vi "procedura configura potenza BANCO 2.vi"(9 "All Data":T3 {"MISURE ALL"."Cluster READ NI"."AI (4-20mA)"."AI 15" format="%#_6f"; "MISURE ALL"."Cluster READ NI"."AI (4-20mA)"."AI 14" format="%#_6f"; "MISURE ALL"."Cluster READ NI"."AI (4-20mA)"."AI 13" format="%#_6f"; "MISURE ALL"."Cluster READ NI"."AI (4-20mA)"."AI 11" format="%#_6f"; "MISURE ALL"."Cluster READ NI"."AI (4-20mA)"."AI 10" format="%#_6f"; "MISURE ALL"."Cluster READ NI"."AI (4-20mA)"."AI 9" format="%#_6f"; "MISURE ALL"."Cluster READ NI"."AI (4-20mA)"."AI 4" format="%#_6f"; "MISURE ALL"."Cluster READ NI"."AI (4-20mA)"."AI 12" format="%#_6f"; "MISURE ALL"."Cluster READ NI"."AI (4-20mA)"."AI 0" format="%#_6f"; "MISURE ALL"."Cluster READ NI"."AI (4-20mA)"."AI 1" format="%#_6f"; "MISURE ALL"."Cluster READ NI"."AI (4-20mA)"."AI 2" format="%#_6f"; "MISURE ALL"."Cluster READ NI"."AI (4-20mA)"."AI 3" format="%#_6f"; "MISURE ALL"."Cluster READ NI"."AI (4-20mA)"."AI 5" format="%#_6f"; "MISURE ALL"."Cluster READ NI"."AI (4-20mA)"."AI 6" format="%#_6f"; "MISURE ALL"."Cluster READ NI"."AI (4-20mA)"."AI 7" format="%#_6f"; "MISURE ALL"."Cluster READ NI"."AI (4-20mA)"."AI 8" format="%#_6f"; "MISURE ALL"."Cluster READ NI"."AI (0-10V)"."AI 31" format="%#_6f"; "MISURE ALL"."Cluster READ NI"."AI (0-10V)"."AI 30" format="%#_6f"; "MISURE ALL"."Cluster READ NI"."AI (0-10V)"."AI 29" format="%#_6f"; "MISURE ALL"."Cluster READ NI"."AI (0-10V)"."AI 28" format="%#_6f"; "MISURE ALL"."Cluster READ NI"."AI (0-10V)"."AI 27" format="%#_6f"; "MISURE ALL"."Cluster READ NI"."AI (0-10V)"."AI 26" format="%#_6f"; "MISURE ALL"."Cluster READ NI"."AI (0-10V)"."AI 25" format="%#_6f"; "MISURE ALL"."Cluster READ NI"."AI (0-10V)"."AI 24" format="%#_6f"; "MISURE ALL"."Cluster READ NI"."AI (0-10V)"."AI 23" format="%#_6f"; "MISURE ALL"."Cluster READ NI"."AI (0-10V)"."AI 22" format="%#_6f"; "MISURE ALL"."Cluster READ NI"."AI (0-10V)"."AI 21" format="%#_6f"; "MISURE ALL"."Cluster READ NI"."AI (0-10V)"."AI 20" format="%#_6f"; "MISURE ALL"."Cluster READ NI"."AI (0-10V)"."AI 19" format="%#_6f"; "MISURE ALL"."Cluster READ NI"."AI (0-10V)"."AI 18" format="%#_6f"; "MISURE ALL"."Cluster READ NI"."AI (0-10V)"."AI 17" format="%#_6f"; "MISURE ALL"."Cluster READ NI"."AI (0-10V)"."AI 16" format="%#_6f"; "MISURE ALL"."Cluster READ NI"."AI (0-10V)"."AI 15" format="%#_6f"; "MISURE ALL"."Cluster READ NI"."AI (0-10V)"."AI 14" format="%#_6f"; "MISURE ALL"."Cluster READ NI"."AI (0-10V)"."AI 13" format="%#_6f"; "MISURE ALL"."Cluster READ NI"."AI (0-10V)"."AI 11" format="%#_6f"; "MISURE ALL"."Cluster READ NI"."AI (0-10V)"."AI 10" format="%#_6f"; "MISURE ALL"."Cluster READ NI"."AI (0-10V)"."AI 9" format="%#_6f"; "MISURE ALL"."Cluster READ NI"."AI (0-10V)"."AI 4" format="%#_6f"; "MISURE ALL"."Cluster READ NI"."AI (0-10V)"."AI 12" format="%#_6f"; "MISURE ALL"."Cluster READ NI"."AI (0-10V)"."AI 0" format="%#_6f"; "MISURE ALL"."Cluster READ NI"."AI (0-10V)"."AI 1" format="%#_6f"; "MISURE ALL"."Cluster READ NI"."AI (0-10V)"."AI 2" format="%#_6f"; "MISURE ALL"."Cluster READ NI"."AI (0-10V)"."AI 3" format="%#_6f"; "MISURE ALL"."Cluster READ NI"."AI (0-10V)"."AI 5" format="%#_6f"; "MISURE ALL"."Cluster READ NI"."AI (0-10V)"."AI 6" format="%#_6f"; "MISURE ALL"."Cluster READ NI"."AI (0-10V)"."AI 7" format="%#_6f"; "MISURE ALL"."Cluster READ NI"."AI (0-10V)"."AI 8" format="%#_6f"}, 10 "Impostazioni elettriche in":T2, 11 "Stato":string) -> (0 "This VI":refnum<vi>, 2 "Boolean":bool, 3 "stato":string)   [LabVIEW 2019]
uses:
  TypeDef/Cluster MISURE.ctl
  TypeDef/MISURE NM.ctl
  TypeDef/Cluster misure ALL.ctl
  TypeDef/Cluster NI.ctl
  cDAQ_PLC Folder/controls/StatoAO_cdaq.ctl
  cDAQ_PLC Folder/controls/statoDO_Cdaq.ctl
  TypeDef/MISURE WT.ctl
  TypeDef/ClusterRes.ctl
  TypeDef/INTERFACCIA.ctl
  TypeDef/Lista AO sistema.ctl
  TypeDef/DOinterfaccia.ctl
  cDAQ_PLC Folder/ST1200_LIST_IO/STATO PLC 1.ctl
  cDAQ_PLC Folder/ST1200_LIST_IO/Uscite PLC 1.ctl
  cDAQ_PLC Folder/controls/statoAO_plc_1.ctl
  cDAQ_PLC Folder/ST1200_LIST_IO/StatoDO_PLC_1.ctl
  SINUS PENTA SANTERNO/controls/Parametri inverter letti.ctl
  cDAQ_PLC Folder/ST1200_LIST_IO/STATO PLC 2.ctl
  cDAQ_PLC Folder/ST1200_LIST_IO/Uscite PLC 2.ctl
  cDAQ_PLC Folder/controls/statoAO_plc_2.ctl
  cDAQ_PLC Folder/ST1200_LIST_IO/StatoDO_PLC_2.ctl
  cDAQ_PLC Folder/ST1200_LIST_IO/STATO PLC 3.ctl
  cDAQ_PLC Folder/ST1200_LIST_IO/Uscite PLC 3.ctl
  cDAQ_PLC Folder/controls/statoAO_plc_3.ctl
  cDAQ_PLC Folder/ST1200_LIST_IO/StatoDO_PLC_3.ctl
  DCREG/Parametri DCREG letti.ctl
  TypeDef/Impostazioni elettriche.ctl
  TypeDef/Collegamenti_elettrici.ctl
  cDAQ_PLC Folder/cDAQ/SET ARRAY DO.ctl
  cDAQ_PLC Folder/cDAQ/SET SINGLE DO.ctl
  cDAQ_PLC Folder/cDAQ/DO List.ctl
  Global allarmi procedure.vi
panel:
  out "COLLEGAMENTO":T1
  out "Stato 2":string
  out "String":string
  # "CONFIGURAZIONE BANCO 2  (KEB)"
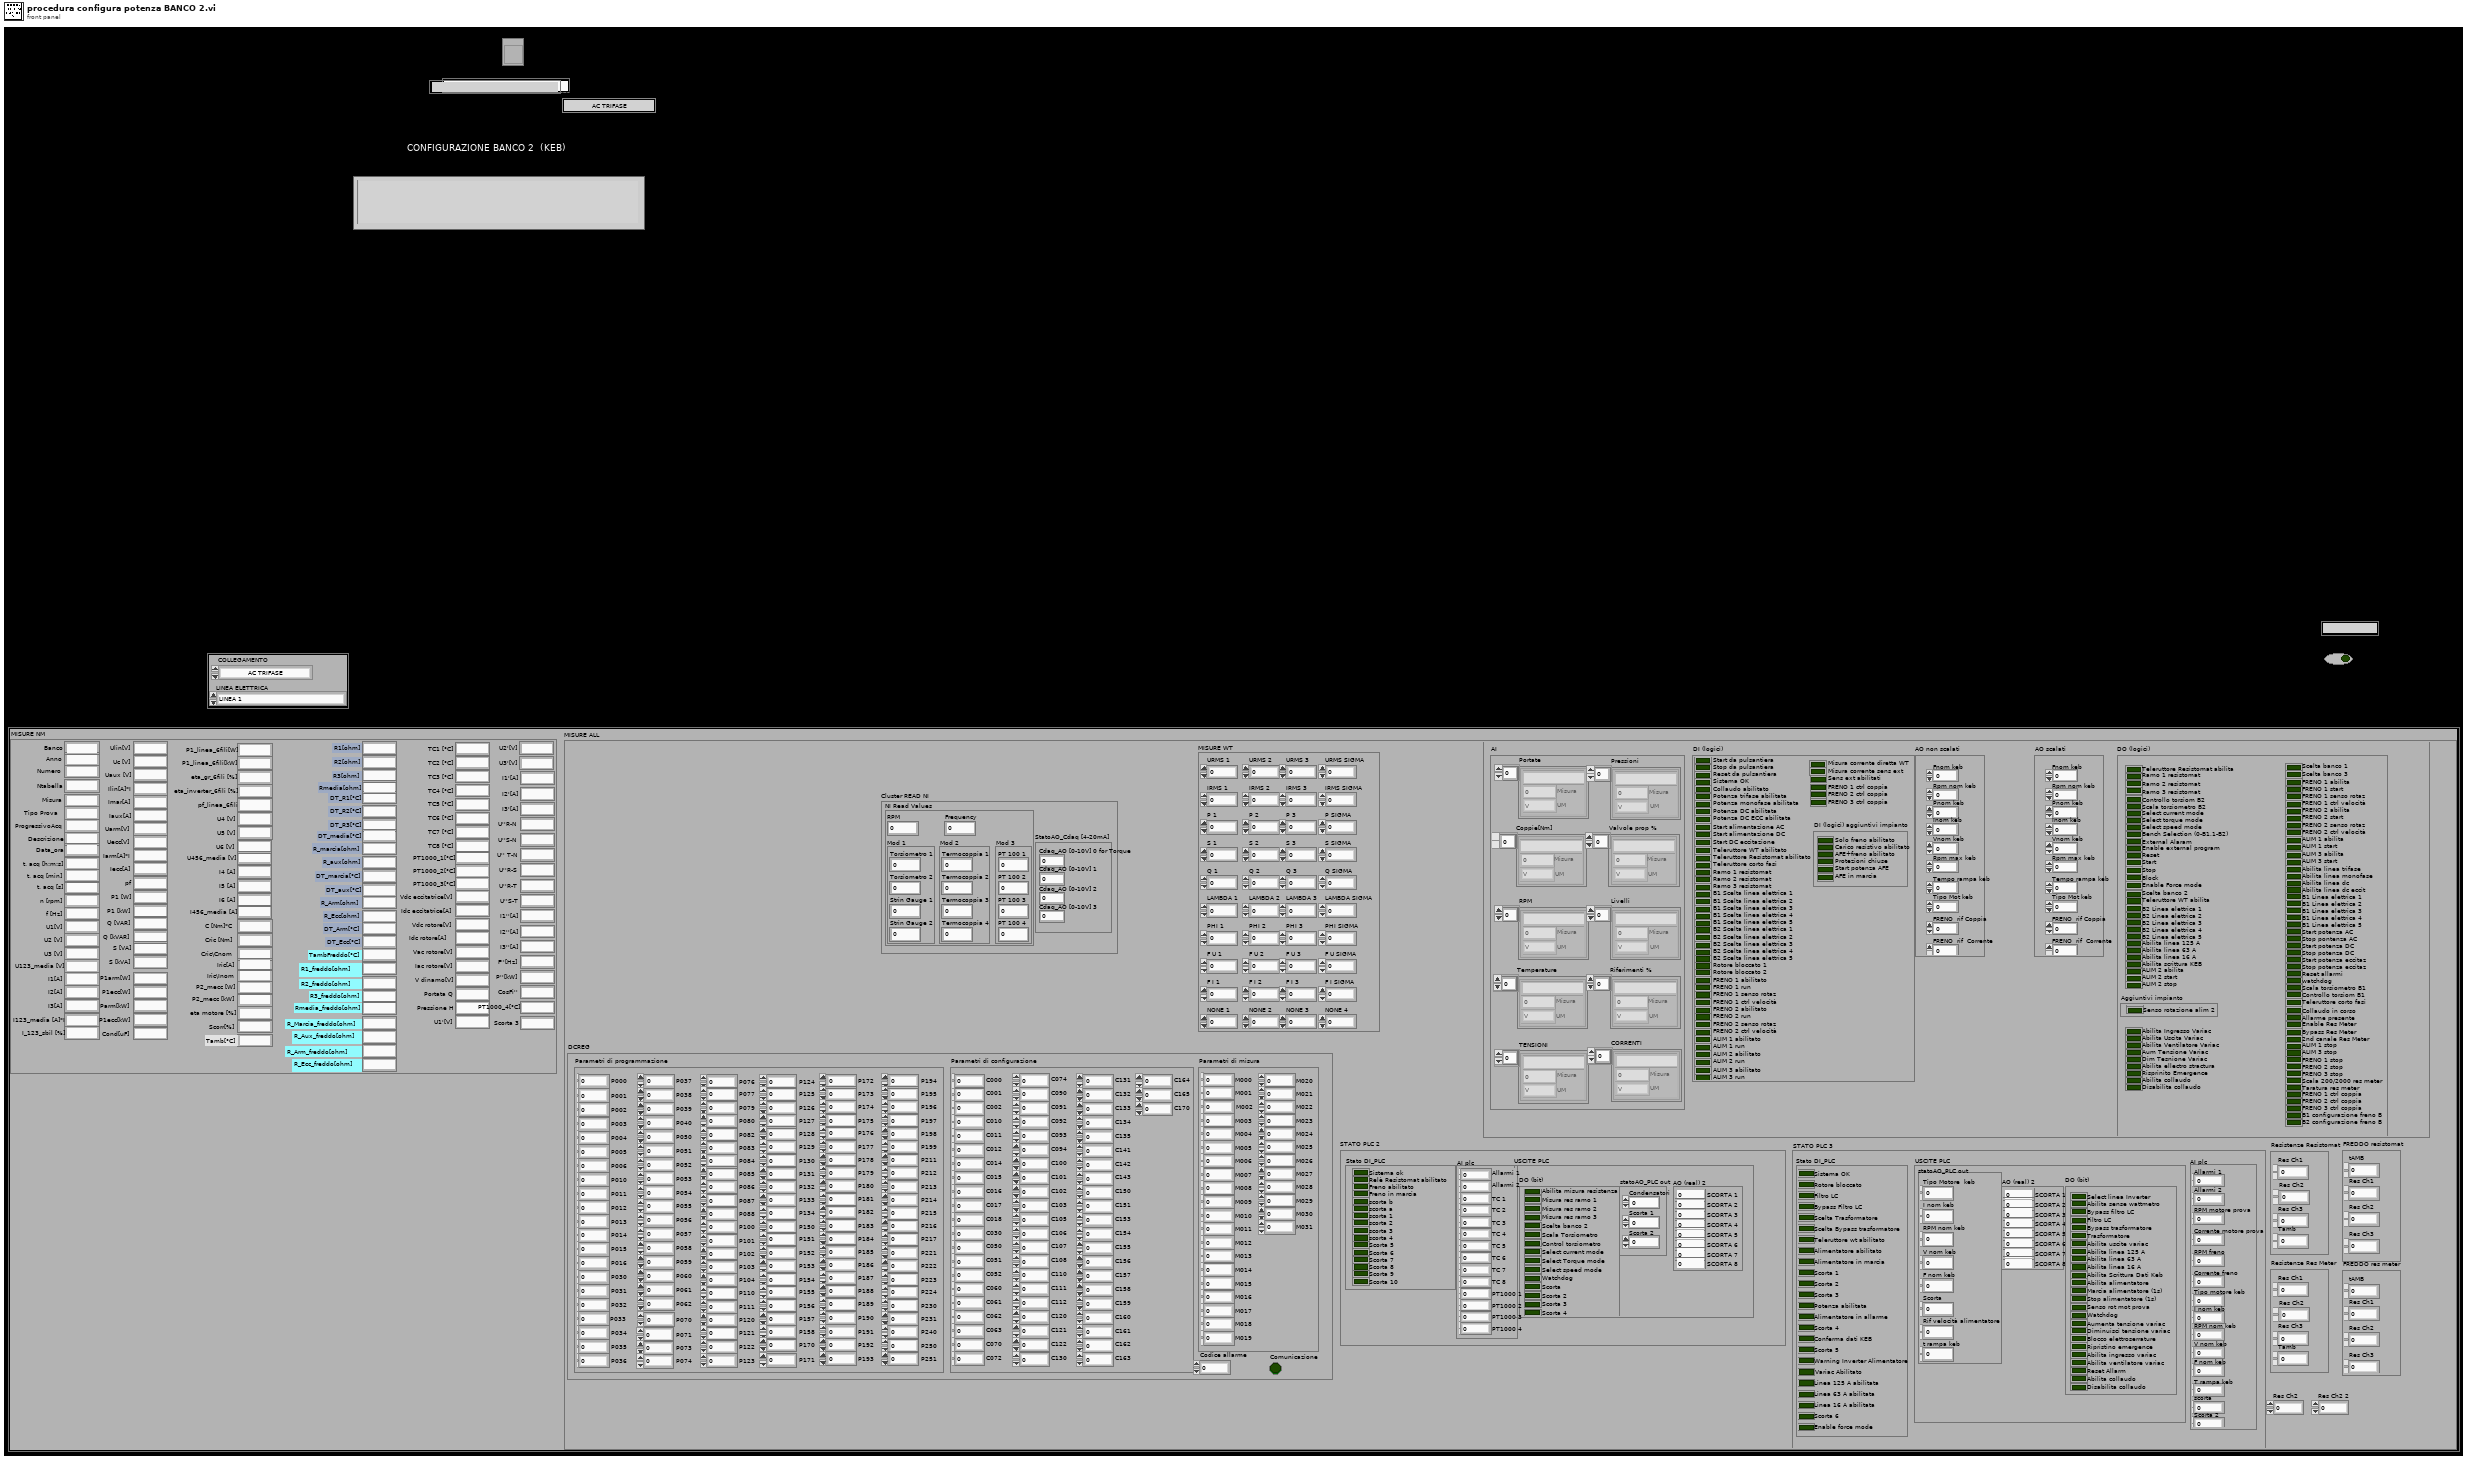
[diagram p1: front panel]
types:
  T1 = typedef "Collegamenti_elettrici.ctl" = enum16{"AC TRIFASE", "AC TRIFASE + FRENO", "AC MONOFASE", "DC CON ECCITAZIONE", "DC CON ECCITAZIONE + FRENO", "DC NO ECCITAZIONE", "DC NO ECCITAZIONE + FRENO", "FRENO TRASC + AFE", "SOLO FRENO", "CARICO RESISTIVO", "GENERICO", "SOLO ACQUISITORE", "SCORTA 4", "SCORTA 5", "SCORTA 6"}
  T2 = typedef "Impostazioni elettriche.ctl" = cluster{"COLLEGAMENTO":T1, "LINEA ELETTRICA":enum16{"LINEA 1", "LINEA 2", "LINEA 3", "LINEA 4", "LINEA 5"}}
  T3 = typedef "Cluster MISURE.ctl" = cluster{"MISURE NM":T4, "MISURE ALL":T5}
  T4 = typedef "MISURE NM.ctl" = cluster{"Banco":string, "Anno":string, "Numero":string, "Ntabella":string, "Misura":string, "Tipo Prova":string, "ProgressivoAcq":string, "Descrizione":string, "Data_ora":string, "t. acq [h:m:s]":string, "t. acq [min]":string, "t. acq [s]":string, "n [rpm]":string, "f [Hz]":string, "U1[V]":string, "U2 [V]":string, "U3 [V]":string, "U123_media [V]":string, "I1[A]":string, "I2[A]":string, "I3[A]":string, "I123_media [A]*I":string, "I_123_sbil [%]":string, "Ulin[V]":string, "Uc [V]":string, "Uaux [V]":string, "Ilin[A]*I":string, "Imar[A]":string, "Iaux[A]":string, "Uarm[V]":string, "Uecc[V]":string, "Iarm[A]*I":string, "Iecc[A]":string, "pf":string, "P1 [W]":string, "P1 [kW]":string, "Q [VAR]":string, "Q [kVAR]":string, "S [VA]":string, "S [kVA]":string, "P1arm[W]":string, "P1ecc[W]":string, "Parm[kW]":string, "P1ecc[kW]":string, "Cond[uF]":string, "P1_linea_6fili[W]":string, "P1_linea_6fili[kW]":string, "eta_gr_6fili [%]":string, "eta_inverter_6fili [%]":string, "pf_linea_6fili":string, "U4 [V]":string, "U5 [V]":string, "U6 [V]":string, "U456_media [V]":string, "I4 [A]":string, "I5 [A]":string, "I6 [A]":string, "I456_media [A]":string, "C [Nm]*C":string, "Cric [Nm]":string, "Cric\\Cnom":string, "Iric[A]":string, "Iric\\Inom":string, "P2_mecc [W]":string, "P2_mecc [kW]":string, "eta motore [%]":string, "Scorr[%]":string, "Tamb[°C]":string, "R1[ohm]":string, "R2[ohm]":string, "R3[ohm]":string, "Rmedia[ohm]":string, "DT_R1[°C]":string, "DT_R2[°C]":string, "DT_R3[°C]":string, "DT_media[°C]":string, "R_marcia[ohm]":string, "R_aux[ohm]":string, "DT_marcia[°C]":string, "DT_aux[°C]":string, "R_Arm[ohm]":string, "R_Ecc[ohm]":string, "DT_Arm[°C]":string, "DT_Ecc[°C]":string, "TambFreddo[°C]":string, "R1_freddo[ohm]":string, "R2_freddo[ohm]":string, "R3_freddo[ohm]":string, "Rmedia_freddo[ohm]":string, "R_Marcia_freddo[ohm]":string, "R_Aux_freddo[ohm]":string, "R_Arm_freddo[ohm]":string, "R_Ecc_freddo[ohm]":string, "TC1 [°C]":string, "TC2 [°C]":string, "TC3 [°C]":string, "TC4 [°C]":string, "TC5 [°C]":string, "TC6 [°C]":string, "TC7 [°C]":string, "TC8 [°C]":string, "PT1000_1[°C]":string, "PT1000_2[°C]":string, "PT1000_3[°C]":string, "Vdc eccitatrice[V]":string, "Idc eccitatrice[A]":string, "Vdc rotore[V]":string, "Idc rotore[A]":string, "Vac rotore[V]":string, "Iac rotore[V]":string, "V dinamo[V]":string, "Portata Q":string, "Pressione H":string, "U1'[V]":string, "U2'[V]":string, "U3'[V]":string, "I1'[A]":string, "I2'[A]":string, "I3'[A]":string, "U''R-N":string, "U''S-N":string, "U'' T-N":string, "U''R-S":string, "U''R-T":string, "U''S-T":string, "I1''[A]":string, "I2''[A]":string, "I3''[A]":string, "F''[Hz]":string, "P''[kW]":string, "CosFi''":string, "PT1000_4[°C]":string, "Scorta 3":string}
  T5 = typedef "Cluster misure ALL.ctl" = cluster{"Cluster READ NI":T6, "MISURE WT":T9, "Resistenze Resistomat":T10, "INTERFACCIA":T11, "FREDDO resistomat":cluster{"Res Ch1":dbl, "Res Ch2":dbl, "tAMB":dbl, "Res Ch3":dbl}, "STATO PLC 1":T16, "Res Ch2":dbl, "Res Ch2 2":dbl, "FREDDO res meter":cluster{"Res Ch1":dbl, "Res Ch2":dbl, "tAMB":dbl, "Res Ch3":dbl}, "Resistenze Res Meter":T10, "READ SINUS PENTA":T20, "STATO PLC 2":T21, "STATO PLC 3":T25, "DCREG":T29}
  T6 = typedef "Cluster NI.ctl" = cluster{"AI (0-10V)":cluster{"AI 0":dbl, "AI 1":dbl, "AI 2":dbl, "AI 3":dbl, "AI 4":dbl, "AI 5":dbl, "AI 6":dbl, "AI 7":dbl, "AI 8":dbl, "AI 9":dbl, "AI 10":dbl, "AI 11":dbl, "AI 12":dbl, "AI 13":dbl, "AI 14":dbl, "AI 15":dbl, "AI 16":dbl, "AI 17":dbl, "AI 18":dbl, "AI 19":dbl, "AI 20":dbl, "AI 21":dbl, "AI 22":dbl, "AI 23":dbl, "AI 24":dbl, "AI 25":dbl, "AI 26":dbl, "AI 27":dbl, "AI 28":dbl, "AI 29":dbl, "AI 30":dbl, "AI 31":dbl}, "StatoAO_Cdaq[0-10V]":cluster{"AO 1":dbl, "AO 2":dbl, "AO 3":dbl, "AO 4":dbl}, "Contatori [rpm]":cluster{"RPM 1":dbl, "RPM 2":dbl}, "StatoAO_Cdaq [4-20mA]":T7, "StatoDO_Cdaq":T8, "DI":cluster{"Scorta 0":bool, "Scorta 1":bool, "Scorta 2":bool, "Scorta 3":bool, "Scorta 4":bool, "Scorta 5":bool, "Scorta 6":bool, "Scorta 7":bool, "Scorta 8":bool, "Scorta 9":bool, "Scorta 10":bool, "Scorta 11":bool, "Scorta 12":bool, "Scorta 13":bool, "Scorta 14":bool, "Scorta 15":bool, "Scorta 16":bool, "Scorta 17":bool, "Scorta 18":bool, "Scorta 19":bool, "Scorta 20":bool, "Scorta 21":bool, "Scorta 22":bool, "Scorta 23":bool, "Scorta 24":bool, "Scorta 25":bool, "Scorta 26":bool, "Scorta 27":bool, "Scorta 28":bool, "Scorta 29":bool, "Scorta 30":bool, "Scorta 31":bool}, "AI (4-20mA)":cluster{"AI 0":dbl, "AI 1":dbl, "AI 2":dbl, "AI 3":dbl, "AI 4":dbl, "AI 5":dbl, "AI 6":dbl, "AI 7":dbl, "AI 8":dbl, "AI 9":dbl, "AI 10":dbl, "AI 11":dbl, "AI 12":dbl, "AI 13":dbl, "AI 14":dbl, "AI 15":dbl}, "TC [°C]":cluster{"tc 1":dbl, "tc 2":dbl, "tc 3":dbl, "tc 4":dbl}, "NI Read Values":cluster{"RPM":dbl, "Frequency":dbl, "Mod 1":cluster{"Torsiometro 1":dbl, "Torsiometro 2":dbl, "Strin Gauge 1":dbl, "Strin Gauge 2":dbl}, "Mod 2":cluster{"Termocoppia 1":dbl, "Termocoppia 2":dbl, "Termocoppia 3":dbl, "Termocoppia 4":dbl}, "Mod 3":cluster{"PT 100 1":dbl, "PT 100 2":dbl, "PT 100 3":dbl, "PT 100 4":dbl}}}
  T7 = typedef "StatoAO_cdaq.ctl" = cluster{"Cdaq_AO [0-10V] 0 for Torque":dbl, "Cdaq_AO [0-10V] 1":dbl, "Cdaq_AO [0-10V] 2":dbl, "Cdaq_AO [0-10V] 3":dbl}
  T8 = typedef "statoDO_Cdaq.ctl" = cluster{"Scorta 0":bool, "Scorta 1":bool, "Scorta 2":bool, "Scorta 3":bool, "Scorta 4":bool, "Scorta 5":bool, "Scorta 6":bool, "Scorta 7":bool, "Scorta 8":bool, "Scorta 9":bool, "Scorta 10":bool, "Scorta 11":bool, "Scorta 12":bool, "Scorta 13":bool, "Scorta 14":bool, "Scorta 15":bool, "Scorta 16":bool, "Scorta 17":bool, "Scorta 18":bool, "Scorta 19":bool, "Scorta 20":bool, "Scorta 21":bool, "Scorta 22":bool, "Scorta 23":bool, "Scorta 24":bool, "Scorta 25":bool, "Scorta 26":bool, "Scorta 27":bool, "Scorta 28":bool, "Scorta 29":bool, "Scorta 30":bool, "Scorta 31":bool}
  T9 = typedef "MISURE WT.ctl" = cluster{"URMS 1":dbl, "IRMS 1":dbl, "P 1":dbl, "S 1":dbl, "Q 1":dbl, "LAMBDA 1":dbl, "PHI 1":dbl, "F U 1":dbl, "F I 1":dbl, "NONE 1":dbl, "URMS 2":dbl, "IRMS 2":dbl, "P 2":dbl, "S 2":dbl, "Q 2":dbl, "LAMBDA 2":dbl, "PHI 2":dbl, "F U 2":dbl, "F I 2":dbl, "NONE 2":dbl, "URMS 3":dbl, "IRMS 3":dbl, "P 3":dbl, "S 3":dbl, "Q 3":dbl, "LAMBDA 3":dbl, "PHI 3":dbl, "F U 3":dbl, "F I 3":dbl, "NONE 3":dbl, "URMS SIGMA":dbl, "IRMS SIGMA":dbl, "P SIGMA":dbl, "S SIGMA":dbl, "Q SIGMA":dbl, "LAMBDA SIGMA":dbl, "PHI SIGMA":dbl, "F U SIGMA":dbl, "F I SIGMA":dbl, "NONE 4":dbl}
  T10 = typedef "ClusterRes.ctl" = cluster{"Res Ch1":dbl, "Res Ch2":dbl, "Res Ch3":dbl, "Tamb":dbl}
  T11 = typedef "INTERFACCIA.ctl" = cluster{"AI":cluster{"Portate":T12[], "Pressioni":T12[], "Coppie[Nm]":T12[], "Valvole prop %":T12[], "RPM":T12[], "Livelli":T12[], "Temperature":T12[], "Riferimenti %":T12[], "TENSIONI":T12[], "CORRENTI":T12[]}, "DI (logici)":cluster{"Start da pulsantiera":bool, "Stop da pulsantiera":bool, "Reset da pulsantiera":bool, "Sistema OK":bool, "Collaudo abilitato":bool, "Potenza trifase abilitata":bool, "Potenza monofase abilitata":bool, "Potenza DC abilitata":bool, "Potenza DC ECC abilitata":bool, "Start alimentazione AC":bool, "Start alimentazione DC":bool, "Start DC eccitazione":bool, "Teleruttore WT abilitato":bool, "Teleruttore Resistomat abilitato":bool, "Teleruttore corto fasi":bool, "Ramo 1 resistomat":bool, "Ramo 2 resistomat":bool, "Ramo 3 resistomat":bool, "B1 Scelta linea elettrica 1":bool, "B1 Scelta linea elettrica 2":bool, "B1 Scelta linea elettrica 3":bool, "B1 Scelta linea elettrica 4":bool, "B1 Scelta linea elettrica 5":bool, "B2 Scelta linea elettrica 1":bool, "B2 Scelta linea elettrica 2":bool, "B2 Scelta linea elettrica 3":bool, "B2 Scelta linea elettrica 4":bool, "B2 Scelta linea elettrica 5":bool, "Rotore bloccato 1":bool, "Rotore bloccato 2":bool, "FRENO 1 abilitato":bool, "FRENO 1 run":bool, "FRENO 1 senso rotaz":bool, "FRENO 1 ctrl velocità":bool, "FRENO 2 abilitato":bool, "FRENO 2 run":bool, "FRENO 2 senso rotaz":bool, "FRENO 2 ctrl velocità":bool, "ALIM 1 abilitato":bool, "ALIM 1 run":bool, "ALIM 2 abilitato":bool, "ALIM 2 run":bool, "ALIM 3 abilitato":bool, "ALIM 3 run":bool, "FRENO 1 ctrl coppia":bool, "FRENO 2 ctrl coppia":bool, "FRENO 3 ctrl coppia":bool, "DI (logici) aggiuntivi impianto":cluster{"Solo freno abilitato":bool, "Carico resistivo abilitato":bool, "AFE+freno abilitato":bool, "Protezioni chiuse":bool, "Start potenza AFE":bool, "AFE in marcia":bool}, "Misura corrente diretta WT":bool, "Misura corrente sens ext":bool, "Sens ext abilitati":bool}, "AO non scalati":T14, "AO scalati":T14, "DO (logici)":T15}
  T12 = typedef "ClusterMisura_e_Unità_INPUT.ctl" = cluster{"Misura":dbl, "UM":T13, "Descrizione":string}
  T13 = typedef "UnitàMisura.ctl" = enum16{"V", "mA", "Bar", "RPM", "m3/s", "m3/min", "m3/h", "l/s", "l/min", "in3/min", "ft3/min", "gpm", "igpm", "igph", "%", "°C", "m", "Nm", "A"}
  T14 = typedef "Lista AO sistema.ctl" = cluster{"FRENO1 rif vel":dbl, "FRENO1 rif Coppia":dbl, "FRENO2 rif vel":dbl, "FRENO2 rif Coppia":dbl, "ALIM1 rif V":dbl, "ALIM1 rif F":dbl, "ALIM2 rif V":dbl, "ALIM2 rif F":dbl, "ALIM3 rif V":dbl, "ALIM3 rif F":dbl, "Fnom keb":dbl, "Rpm nom keb":dbl, "Pnom keb":dbl, "Inom keb":dbl, "Vnom keb":dbl, "Rpm max keb":dbl, "Tempo rampa keb":dbl, "Tipo Mot keb":dbl, "FRENO  rif Coppia ":dbl, "FRENO  rif  Corrente":dbl}
  T15 = typedef "DOinterfaccia.ctl" = cluster{"Scelta banco 1":bool, "Scelta banco 2":bool, "Scelta banco 3":bool, "FRENO 1 abilita":bool, "FRENO 1 start":bool, "FRENO 1 senso rotaz":bool, "FRENO 1 ctrl velocità":bool, "FRENO 2 abilita":bool, "FRENO 2 start":bool, "FRENO 2 senso rotaz":bool, "FRENO 2 ctrl velocità":bool, "ALIM 1 abilita":bool, "ALIM 1 start":bool, "ALIM 2 abilita":bool, "ALIM 2 start":bool, "ALIM 3 abilita":bool, "ALIM 3 start":bool, "Abilita linea trifase":bool, "Abilita linea monofase":bool, "Abilita linea dc":bool, "Abilita linea dc eccit":bool, "B1 Linea elettrica 1":bool, "B1 Linea elettrica 2":bool, "B1 Linea elettrica 3":bool, "B1 Linea elettrica 4":bool, "B1 Linea elettrica 5":bool, "B2 Linea elettrica 1":bool, "B2 Linea elettrica 2":bool, "B2 Linea elettrica 3":bool, "B2 Linea elettrica 4":bool, "B2 Linea elettrica 5":bool, "Start potenza AC":bool, "Stop pontenza AC":bool, "Start potenza DC":bool, "Stop potenza DC":bool, "Start potenza eccitaz":bool, "Stop potenza eccitaz":bool, "Reset allarmi":bool, "watchdog":bool, "Scala torsiometro B1":bool, "Controllo torsiom B1":bool, "Scala torsiometro B2":bool, "Controllo torsiom B2":bool, "Teleruttore WT abilita":bool, "Teleruttore Resistomat abilita":bool, "Teleruttore corto fasi":bool, "Ramo 1 resistomat":bool, "Ramo 2 resistomat":bool, "Ramo 3 resistomat":bool, "Collaudo in corso":bool, "Allarme presente":bool, "Enable Res Meter":bool, "Bypass Res Meter":bool, "2nd canale Res Meter":bool, "Scala 200/2000 res meter":bool, "Taratura res meter":bool, "FRENO 1 ctrl coppia":bool, "FRENO 2 ctrl coppia":bool, "FRENO 3 ctrl coppia":bool, "Aggiuntivi impianto":cluster{"Senso rotazione alim 1":bool, "Senso rotazione alim 2":bool}, "ALIM 1 stop":bool, "ALIM 2 stop":bool, "ALIM 3 stop":bool, "FRENO 1 stop":bool, "FRENO 2 stop":bool, "FRENO 3 stop":bool, "B1 configurazione freno B":bool, "B2 configurazione freno B":bool, "Abilita scrittura KEB":bool, "Bench Selection (0-B1,1-B2)":bool, "Select current mode":bool, "Select torque mode":bool, "Select speed mode":bool, "Start":bool, "Stop":bool, "Block":bool, "Enable Force mode":bool, "Abilita linea 125 A":bool, "Abilita linea 63 A":bool, "Abilita linea 16 A":bool, "Aum Tensione Variac":bool, "Dim Tesnione Variac":bool, "Abilita ellectro stractura":bool, "Risprinito Emergence":bool, "Abilita collaudo":bool, "Disabilita collaudo":bool, "External Alaram":bool, "Enable external program":bool, "Reset":bool, "Abilita Ingresso Variac":bool, "Abilita Ventilatore Variac":bool, "Abilita Uscita Variac ":bool}
  T16 = typedef "STATO PLC 1.ctl" = cluster{"USCITE PLC":T17, "Stato DI_PLC":cluster{"Sistema OK":bool, "Rotore bloccato":bool, "Scorta 1":bool, "Prova diretto inverter":bool, "Prova con filtro LC":bool, "Teleruttore WT abilitato":bool, "Alim sinus penta abilitato":bool, "Alim sinus penta in marcia":bool, "Freno abilitato":bool, "Freno in marcia":bool, "Senso rotazione freno":bool, "Potenza abilitata":bool, "Scorta 3":bool, "Scorta 4":bool, "scorta 5":bool, "scorta 6":bool}, "AI plc":cluster{"Allarmi 1":dbl, "Allarmi 2":dbl, "Scorta 1":dbl, "Scorta 2":dbl, "RPM mot prova":dbl, "I mot prova":dbl, "RPM freno":dbl, "I freno":dbl, "Scorta 3":dbl, "Scorta 4":dbl}}
  T17 = typedef "Uscite PLC 1.ctl" = cluster{"AO (real) 2":cluster{"SCORTA 1":dbl, "SCORTA 2":dbl, "SCORTA 3":dbl, "SCORTA 4":dbl, "SCORTA 5":dbl, "SCORTA 6":dbl, "SCORTA 7":dbl, "SCORTA 8":dbl}, "statoAO_PLC out":T18, "DO (bit)":T19}
  T18 = typedef "statoAO_plc_1.ctl" = cluster{"Rif Lim coppia freno [%]":dbl, "Rif rpm freno [%]":dbl, "Rif coppia freno [%]":dbl, "Rif V alimentatore [%]":dbl, "Rif F alimentatore [%]":dbl}
  T19 = typedef "StatoDO_PLC_1.ctl" = cluster{"Scelta banco 1":bool, "Set dati motore freno 2":bool, "Diretto inverter":bool, "Filtro LC":bool, "Marcia ALIM (1s)":bool, "Marcia FRENO (1s)":bool, "Stop AFE (1s)":bool, "Stop freno (1s)":bool, "Reset allarmi":bool, "Watchdog":bool, "Senso rotazione":bool, "Abilita collaudo (1s)":bool, "Disabilita collaudo (1s)":bool, "Abilitazione ALIM":bool, "Abilitazione FRENO":bool, "Teleruttore WT":bool, "Senso rot motore prova":bool, "Scorta 7":bool, "Scorta 8":bool, "Scorta 9":bool, "Scorta 10":bool, "Scorta 11":bool, "Scorta 12":bool, "Scorta 13":bool}
  T20 = typedef "Parametri inverter letti.ctl" = cluster{"Menù Misure motore (M000-M030)":cluster{"Rif vel a regime (int)":u16, "Rif vel a regime (dec)":u16, "Rif vel dopo rampe (int)":u16, "Rif vel dopo rampe (dec)":u16, "RPM motore (int)":u16, "RPM motore (dec)":u16, "FREQout inverter":u16, "Rif coppia a regime(Nm)":u16, "Richiesta di coppia (Nm)":u16, "Coppia generata dal motore(Nm)":u16, "Rif coppia a regime(%)":u16, "Richiesta di coppia (%)":u16, "Coppia generata dal motore(%)":u16, "Coppia max richiesta prima delle rampe(Nm)":u16, "Coppia max richiesta dopo le rampe(Nm)":u16, "Limite di velocità prima delle rampe":u16, "Limite di velocità dopo le rampe":u16, "Coppia max richiesta prima delle rampe(%)":u16, "Coppia max richiesta dopo le rampe(%)":u16, "Rif di flusso":u16, "Corrente di uscita":u16, "Capacità termica del motore":u16, "Tensione di uscita":u16, "Potenza di uscita":u16, "Energia consumata (LSword)":u16, "Energia consumata (MSword)":u16, "Tensione bus DC":u16, "Tensione di rete":u16}, "Menù regolatore PID (M018-M024)":cluster{"Rif PID a regime(%)":u16, "Rif pid dopo rampe(%)":u16, "Retroazione del pid(%)":u16, "Errore del pid(%)":u16, "uscita del pid(%)":u16, "Rif del pid dopo le rampe":u16, "Retroazione del pid":u16}, "Menù ingressi digitali (M031-M036)":cluster{"Ingressi digitali ritardati":u16, "Ingressi digitali istantanei":u16, "Moresettiera comando loc":u16, "Morsett comando da seriale":u16, "Morsett comando bus di campo":u16, "Ing dig ausiliari da morsettiera":u16, "Ing dig ausiliari da seriale":u16}, "Menù riferimenti (M037-M051)":cluster{"Rif analog est REF":u16, "Rif analog est AIN1":u16, "Rif analog est AIN2":u16, "Rif analog est XAIN4":u16, "Rif analog est XAIN5":u16, "Rif velocità da seriale(int)":u16, "Rif velocità bus di campo(int)":u16, "Rif coppia da seriale":u16, "Rif coppia bus di campo":u16, "Rif del PID da seriale":u16, "Rif del PID da bus di campo":u16, "Retroazione del PID da seriale":u16, "Retroazione del PIDda bus di campo":u16, "Rif da encoder":u16, "Rif in frequenza":u16, "Rif velocità da seriale(dec)":u16, "Rif velocità bus di campo(dec)":u16}, "Menù rampe (P009-P033)":cluster{"Tempo di dec rampa di vel 1":u16, "Tempo di acc rampa di vel 2":u16, "Tempo di dec rampa di vel 2":u16, "Tempo di acc rampa di vel 1":u16, "Unità di mis tempi rampe vel 1/2":u16, "Tempo di acc rampa di vel 3":u16, "Tempo di dec rampa di vel 3":u16, "Tempo di acc rampa di vel 4":u16, "Tempo di dec rampa di vel 4":u16, "Unità di mis tempi rampe vel 3/4":u16, "Selettore arrottondam rampe":u16, "Tempo di arrotond iniz rampa acc":u16, "Tempo di arrotond finale rampa acc":u16, "Tempo di arrotond iniz rampa dec":u16, "Tempo di rampa di salita rif coppia":u16, "Tempo di rampa di discesa rif coppia":u16, "Unità di misura rampa coppia":u16, "Tempo rampa acc marcia jog":u16, "Tempo rampa dec marcia jog":u16, "Reset acc ai cambi pendenza":u16, "rampa di acc in fire mode":u16, "rampa di dec in fire mode":u16, "Tempo di arrotond finale rampa dec":u16}, "Menù controllo motore(C008-C128)":cluster{"Numero motori configurati":u16, "Tipo algoritmo di controllo Mot1":u16, "Tipo rif Mot1":u16, "Tensione nominale rete":u16, "Retroaz di vel da encoder Mot1":u16, "Tipo curva V/f Mot1":u16, "Rotazione delle fasi Mot1":u16, "Freq nominale del motore Mot1":u16, "RPM nominali del motore Mot1":u16, "Potenza nominale del motore Mot1":u16, "Corrente nominale del motore Mot1":u16, "Tensione nominale del motore mot1":u16, "Potenza a vuoto del motore Mot1":u16, "Corrente a vuoto del motore Mot1":u16, "Resistenza statorica del motore Mot1":u16, "Induttanza di dispersione Mot1":u16, "Induttanza mutua motore":u16, "Costante di tempo rotorica":u16, "Costante di tempo filtro pb":u16, "Velocità minima motore":u16, "Velocità massima motore":u16}, "Menù configurazione PID":cluster{"Selezione riferimento n.1":u16, "Selezione retroazione n.1":u16, "Modalità di fuzionamento PID":u16, "Termine derivativo calcolato su err o mis":u16, "Proporz moltiplica deriv e integrale":u16, "Azione del PID":u16}, "ID":dbl, "Menù uscite digitali":cluster{"MDO4 Inverter pronto":u16}, "Fcarrier":cluster{"Fcarrier Min (Hz)":u16, "Fcarrier Max (Hz)":u16}, "stato inverter M089":dbl, "Riferimenti":cluster{"Rif tensione":u16, "Rif velocità":u16}, "Comunicazione":bool, "Modalità stop":dbl}
  T21 = typedef "STATO PLC 2.ctl" = cluster{"USCITE PLC":T22, "Stato DI_PLC":cluster{"Sistema ok":bool, "Relè Resistomat abilitato":bool, "Freno abilitato":bool, "Freno in marcia":bool, "scorta b":bool, "scorta a":bool, "scorta 1":bool, "scorta 2":bool, "scorta 3":bool, "scorta 4":bool, "Scorta 5":bool, "Scorta 6":bool, "Scorta 7":bool, "Scorta 8":bool, "Scorta 9":bool, "Scorta 10":bool}, "AI plc":cluster{"Allarmi 1":dbl, "Allarmi 2":dbl, "TC 1":dbl, "TC 2":dbl, "TC 3":dbl, "TC 4":dbl, "TC 5":dbl, "TC 6":dbl, "TC 7":dbl, "TC 8":dbl, "PT1000 1":dbl, "PT1000 2":dbl, "PT1000 3":dbl, "PT1000 4":dbl}}
  T22 = typedef "Uscite PLC 2.ctl" = cluster{"AO (real) 2":cluster{"SCORTA 1":dbl, "SCORTA 2":dbl, "SCORTA 3":dbl, "SCORTA 4":dbl, "SCORTA 5":dbl, "SCORTA 6":dbl, "SCORTA 7":dbl, "SCORTA 8":dbl}, "statoAO_PLC out":T23, "DO (bit)":T24}
  T23 = typedef "statoAO_plc_2.ctl" = cluster{"Condensatori":dbl, "Scorta 1":dbl, "Scorta 2":dbl}
  T24 = typedef "StatoDO_PLC_2.ctl" = cluster{"Relè misura resistomat":bool, "Misura res ramo 1":bool, "Misura res ramo 2":bool, "Misura res ramo 3":bool, "Scelta banco 2":bool, "Scala Torsiometro":bool, "Ctrl torsiometro":bool, "Select current mode":bool, "Select Torque mode":bool, "Select speed mode":bool, "Watchdog":bool, "Scorta":bool, "Scorta 2":bool, "Scorta 3":bool, "Scorta 4":bool, "Scorta 5":bool, "Bench selection":bool, "External alarm":bool, "Enable external program":bool, "Reset allarmi":bool, "Start":bool, "Stop":bool, "Block":bool, "Scorta 6":bool}
  T25 = typedef "STATO PLC 3.ctl" = cluster{"USCITE PLC":T26, "Stato DI_PLC":cluster{"Sistema OK":bool, "Rotore bloccato":bool, "Filtro LC":bool, "Bypass Filtro LC":bool, "Scelta Trasformatore":bool, "Scelta Bypass trasformatore":bool, "Teleruttore wt abilitato":bool, "Alimentatore abilitato":bool, "Alimentatore in marcia":bool, "Scorta 1":bool, "Scorta 2":bool, "Scorta 3":bool, "Potenza abilitata":bool, "Alimentatore in allarme":bool, "Scorta 4":bool, "Conferma dati KEB":bool, "Scorta 5":bool, "Warning Inverter Alimentatore":bool, "Variac Abilitato":bool, "Linea 125 A abilitata":bool, "Linea 63 A abilitata":bool, "Linea 16 A abilitata":bool, "Scorta 6":bool, "Enable force mode":bool}, "AI plc":cluster{"Allarmi 1":dbl, "Allarmi 2":dbl, "RPM motore prova":dbl, "Corrente motore prova":dbl, "RPM freno":dbl, "Corrente freno":dbl, "Tipo motore keb":dbl, "I nom keb":dbl, "RPM nom keb":dbl, "V nom keb":dbl, "F nom keb":dbl, "T rampa keb":dbl, "scorta":dbl, "Scorta 2":dbl}}
  T26 = typedef "Uscite PLC 3.ctl" = cluster{"AO (real) 2":cluster{"SCORTA 1":dbl, "SCORTA 2":dbl, "SCORTA 3":dbl, "SCORTA 4":dbl, "SCORTA 5":dbl, "SCORTA 6":dbl, "SCORTA 7":dbl, "SCORTA 8":dbl}, "statoAO_PLC out":T27, "DO (bit)":T28}
  T27 = typedef "statoAO_plc_3.ctl" = cluster{"Rif velocità alimentatore":dbl, "Scorta":dbl, "Tipo Motore  keb":dbl, "I nom keb":dbl, "RPM nom keb":dbl, "V nom keb":dbl, "F nom keb":dbl, "t rampa keb":dbl}
  T28 = typedef "StatoDO_PLC_3.ctl" = cluster{"Select linea Inverter":bool, "Abilita sense wattmetro":bool, "Bypass filtro LC":bool, "Filtro LC":bool, "Bypass trasformatore":bool, "Trasformatore":bool, "Abilita uscite variac":bool, "Abilita linea 125 A":bool, "Abilita linea 63 A":bool, "Abilita linea 16 A":bool, "Abilita Scrittura Dati Keb":bool, "Abilita alimentatore":bool, "Marcia alimentatore (1s)":bool, "Stop alimentatore (1s)":bool, "Senso rot mot prova":bool, "Watchdog":bool, "Aumenta tensione variac":bool, "Diminuisci tensione variac ":bool, "Blocco elettroserrature":bool, "Ripristino emergence":bool, "Abilita ingresso variac":bool, "Abilita ventilatore variac":bool, "Reset Allarm":bool, "Scorta 1":bool, "Scorta 2":bool, "Scorta 3":bool, "Scorta 4":bool, "Scorta 5":bool, "Scorta 6":bool, "Scorta 7":bool, "Scorta 8":bool, "Scorta 9":bool, "Abilita collaudo":bool, "Disabilita collaudo ":bool, "Scorta 10":bool, "Scorta 11":bool, "Scorta 12":bool, "Scorta 13":bool, "Scorta 14":bool, "Scorta 15":bool}
  T29 = typedef "Parametri DCREG letti.ctl" = cluster{"Parametri di misura":cluster{"M000":dbl, "M001":dbl, "M002":dbl, "M003":dbl, "M004":dbl, "M005":dbl, "M006":dbl, "M007":dbl, "M008":dbl, "M009":dbl, "M010":dbl, "M011":dbl, "M012":dbl, "M013":dbl, "M014":dbl, "M015":dbl, "M016":dbl, "M017":dbl, "M018":dbl, "M019":dbl, "M020":dbl, "M021":dbl, "M022":dbl, "M023":dbl, "M024":dbl, "M025":dbl, "M026":dbl, "M027":dbl, "M028":dbl, "M029":dbl, "M030":dbl, "M031":dbl}, "Parametri di programmazione":cluster{"P000":dbl, "P001":dbl, "P002":dbl, "P003":dbl, "P004":dbl, "P005":dbl, "P006":dbl, "P010":dbl, "P011":dbl, "P012":dbl, "P013":dbl, "P014":dbl, "P015":dbl, "P016":dbl, "P030":dbl, "P031":dbl, "P032":dbl, "P033":dbl, "P034":dbl, "P035":dbl, "P036":dbl, "P037":dbl, "P038":dbl, "P039":dbl, "P040":dbl, "P050":dbl, "P051":dbl, "P052":dbl, "P053":dbl, "P054":dbl, "P055":dbl, "P056":dbl, "P057":dbl, "P058":dbl, "P059":dbl, "P060":dbl, "P061":dbl, "P062":dbl, "P070":dbl, "P071":dbl, "P073":dbl, "P074":dbl, "P076":dbl, "P077":dbl, "P079":dbl, "P080":dbl, "P082":dbl, "P083":dbl, "P084":dbl, "P085":dbl, "P086":dbl, "P087":dbl, "P088":dbl, "P100":dbl, "P101":dbl, "P102":dbl, "P103":dbl, "P104":dbl, "P110":dbl, "P111":dbl, "P120":dbl, "P121":dbl, "P122":dbl, "P123":dbl, "P124":dbl, "P125":dbl, "P126":dbl, "P127":dbl, "P128":dbl, "P129":dbl, "P130":dbl, "P131":dbl, "P132":dbl, "P133":dbl, "P134":dbl, "P150":dbl, "P151":dbl, "P152":dbl, "P153":dbl, "P154":dbl, "P155":dbl, "P156":dbl, "P157":dbl, "P158":dbl, "P170":dbl, "P171":dbl, "P172":dbl, "P173":dbl, "P174":dbl, "P175":dbl, "P176":dbl, "P177":dbl, "P178":dbl, "P179":dbl, "P180":dbl, "P181":dbl, "P182":dbl, "P183":dbl, "P184":dbl, "P185":dbl, "P186":dbl, "P187":dbl, "P188":dbl, "P189":dbl, "P190":dbl, "P191":dbl, "P192":dbl, "P193":dbl, "P194":dbl, "P195":dbl, "P196":dbl, "P197":dbl, "P198":dbl, "P199":dbl, "P211":dbl, "P212":dbl, "P213":dbl, "P214":dbl, "P215":dbl, "P216":dbl, "P217":dbl, "P221":dbl, "P222":dbl, "P223":dbl, "P224":dbl, "P230":dbl, "P231":dbl, "P240":dbl, "P250":dbl, "P251":dbl}, "Parametri di configurazione":cluster{"C000":dbl, "C001":dbl, "C002":dbl, "C010":dbl, "C011":dbl, "C012":dbl, "C014":dbl, "C015":dbl, "C016":dbl, "C017":dbl, "C018":dbl, "C030":dbl, "C050":dbl, "C051":dbl, "C052":dbl, "C060":dbl, "C061":dbl, "C062":dbl, "C063":dbl, "C070":dbl, "C072":dbl, "C074":dbl, "C090":dbl, "C091":dbl, "C092":dbl, "C093":dbl, "C094":dbl, "C100":dbl, "C101":dbl, "C102":dbl, "C103":dbl, "C105":dbl, "C106":dbl, "C107":dbl, "C108":dbl, "C110":dbl, "C111":dbl, "C112":dbl, "C120":dbl, "C121":dbl, "C122":dbl, "C130":dbl, "C131":dbl, "C132":dbl, "C133":dbl, "C134":dbl, "C135":dbl, "C141":dbl, "C142":dbl, "C143":dbl, "C150":dbl, "C151":dbl, "C153":dbl, "C154":dbl, "C155":dbl, "C156":dbl, "C157":dbl, "C158":dbl, "C159":dbl, "C160":dbl, "C161":dbl, "C162":dbl, "C163":dbl, "C164":dbl, "C165":dbl, "C170":dbl}, "Codice allarme":dbl, "Comunicazione":bool}
  T30 = enum16{"LINEA 1", "LINEA 2", "LINEA 3", "LINEA 4", "LINEA 5"}
  T31 = cluster{"Start da pulsantiera":bool, "Stop da pulsantiera":bool, "Reset da pulsantiera":bool, "Sistema OK":bool, "Collaudo abilitato":bool, "Potenza trifase abilitata":bool, "Potenza monofase abilitata":bool, "Potenza DC abilitata":bool, "Potenza DC ECC abilitata":bool, "Start alimentazione AC":bool, "Start alimentazione DC":bool, "Start DC eccitazione":bool, "Teleruttore WT abilitato":bool, "Teleruttore Resistomat abilitato":bool, "Teleruttore corto fasi":bool, "Ramo 1 resistomat":bool, "Ramo 2 resistomat":bool, "Ramo 3 resistomat":bool, "B1 Scelta linea elettrica 1":bool, "B1 Scelta linea elettrica 2":bool, "B1 Scelta linea elettrica 3":bool, "B1 Scelta linea elettrica 4":bool, "B1 Scelta linea elettrica 5":bool, "B2 Scelta linea elettrica 1":bool, "B2 Scelta linea elettrica 2":bool, "B2 Scelta linea elettrica 3":bool, "B2 Scelta linea elettrica 4":bool, "B2 Scelta linea elettrica 5":bool, "Rotore bloccato 1":bool, "Rotore bloccato 2":bool, "FRENO 1 abilitato":bool, "FRENO 1 run":bool, "FRENO 1 senso rotaz":bool, "FRENO 1 ctrl velocità":bool, "FRENO 2 abilitato":bool, "FRENO 2 run":bool, "FRENO 2 senso rotaz":bool, "FRENO 2 ctrl velocità":bool, "ALIM 1 abilitato":bool, "ALIM 1 run":bool, "ALIM 2 abilitato":bool, "ALIM 2 run":bool, "ALIM 3 abilitato":bool, "ALIM 3 run":bool, "FRENO 1 ctrl coppia":bool, "FRENO 2 ctrl coppia":bool, "FRENO 3 ctrl coppia":bool, "DI (logici) aggiuntivi impianto":cluster{"Solo freno abilitato":bool, "Carico resistivo abilitato":bool, "AFE+freno abilitato":bool, "Protezioni chiuse":bool, "Start potenza AFE":bool, "AFE in marcia":bool}, "Misura corrente diretta WT":bool, "Misura corrente sens ext":bool, "Sens ext abilitati":bool}
  T32 = typedef "SET ARRAY DO.ctl" = T33[]
  T33 = typedef "SET SINGLE DO.ctl" = cluster{"DO":T34, "Value":bool}
  T34 = typedef "DO List.ctl" = enum16{"OFF: ALL DO", "*ABILITA freno 1", "*ABILITA freno 2", "*ABILITA freno 3", "*START freno 1", "*START freno 2", "*START freno 3", "*STOP freno 1", "*STOP freno 3", "*STOP freno 2", "*Senso rot freno 1", "*Senso rot freno 2", "*Senso rot freno 3", "*Ctrl velocità freno 1", "*Ctrl velocità freno 2", "*Ctrl velocità freno 3", "*Ctrl coppia freno 1", "*Ctrl coppia freno 2", "*Ctrl coppia freno 3", "*ABILITA alimentatore 1", "*ABILITA alimentatore 2", "*ABILITA alimentatore 3", "*ABILITA alimentatore 4", "*START alimentatore 1", "*START alimentatore 2", "*START alimentatore 3", "*START alimentatore 4", "*STOP alimentatore 1", "*STOP alimentatore 2", "*STOP alimentatore 3", "*STOP alimentatore 4", "SENSO ROT alimentatore 1", "SENSO ROT alimentatore 2", "Abilita LEM 1000A", "Abilita LEM 300A", "Abilita sensori EXT WT", "B1 Seleziona linea 1", "B1 Seleziona linea 2", "B1 Seleziona linea 3", "B1 Seleziona linea 4", "B1 Seleziona linea 5", "B2 Seleziona linea 1", "B2 Seleziona linea 2", "B2 Seleziona linea 3", "B2 Seleziona linea 4", "B2 Seleziona linea 5", "*Reset allarmi", "*Start potenza AC", "*Stop potenza AC", "*Start potenza DC", "*Stop potenza DC", "*Start potenza DC eccit", "*Stop pontenza DC eccit", "Bypass res meter", "2nd canale res meter", "Enable res meter", "*Abilit teler ramo WT", "*Abil teler ramo princ Resit", "*Abil teler ramo 1 Resist", "*Abil teler ramo 2 Resist", "*Abil teler ramo 3 Resist", "*Abil cortocirc avvolgim", "*Controllo torsiometro B1", "*Controllo Torsiom B2", "*Scala torsiometro B1", "*Scala torsiometro B2", "*Collaudo in corso", "*Allarme presente", "Abilitazione elettroserratura", "Exit", "*Abilita collaudo", "*Abilita potenza trifase", "*Abilita potenza monofase", "*Abilita potenza DC", "*Abilita potenza DC eccit", "*Disabilita teleruttori potenza", "Set teleruttori prova a freddo", "Prova a freddo monofase", "Watchdog", "Forza DO PLC 3", "Forza DO PLC 2", "Forza DO PLC 1", "Forza DO cDAQ", "Scala 2000(T) 200(F) res meter", "Seleziona banco 1", "Seleziona banco 2", "Comando azionam in blocco", "Comando azionam reset", "Sensibilità freno 16 32 nm", "Reset Allarmi", "Carico res - Ramo 1", "Carico res - Ramo 2", "Carico res - Ramo 3", "Carico res - Ramo 4", "Carico res - Ramo 5", "Carico res - Ramo 6", "Carico res - Ramo 7", "Carico res - Ramo 8", "Carico res - Ramo 9", "Carico res - Ramo 10", "Carico res - Ramo 11", "Carico res - Start ventilatore", "Carico res - Stop ventilatore", "Abilita potenza solo freno", "Abilita AFE + freno trasc", "Abilita potenza carico resistivo", "Chiudi potenza AFE", "Apri potenza AFE", "Start AFE", "Config Banco2 TDE", "Misura diretto WT", "Ripristina centralina protezioni", "Abilita Scrittura Dati Keb", "Bench Selection(0-B1,1-B2)", "Select current mode", "Select torque mode", "Select speed mode", "Extenal alarm", "Enable Extenal program ", "Start ", "Stop", "Enable force mode", "Abilita linea 125 A", "Abilita linea 63 A", "Abilita linea 16 A", "Aum Tensione Variac", "Dim Tesnione Variac", "Abilita Ellecto Stractura", "Riprinto Emergenxe ", "Abilita Collaudo", "Disabilita Collaudo", "Abilita Ingresso Variac", "Abilita Uscita Variac", "Abilita ventilatore Variac"}
  T35 = enum32{"Invalid", "Standard", "Closed", "Hidden", "Minimized", "Maximized"}
  T36 = cluster{"Array of elements":cluster{"String":string, "variant":variant}[], "Single element":cluster{"String":string, "variant":variant}, "enque at\nopposite end (F)":bool, "no replications (F)":bool}
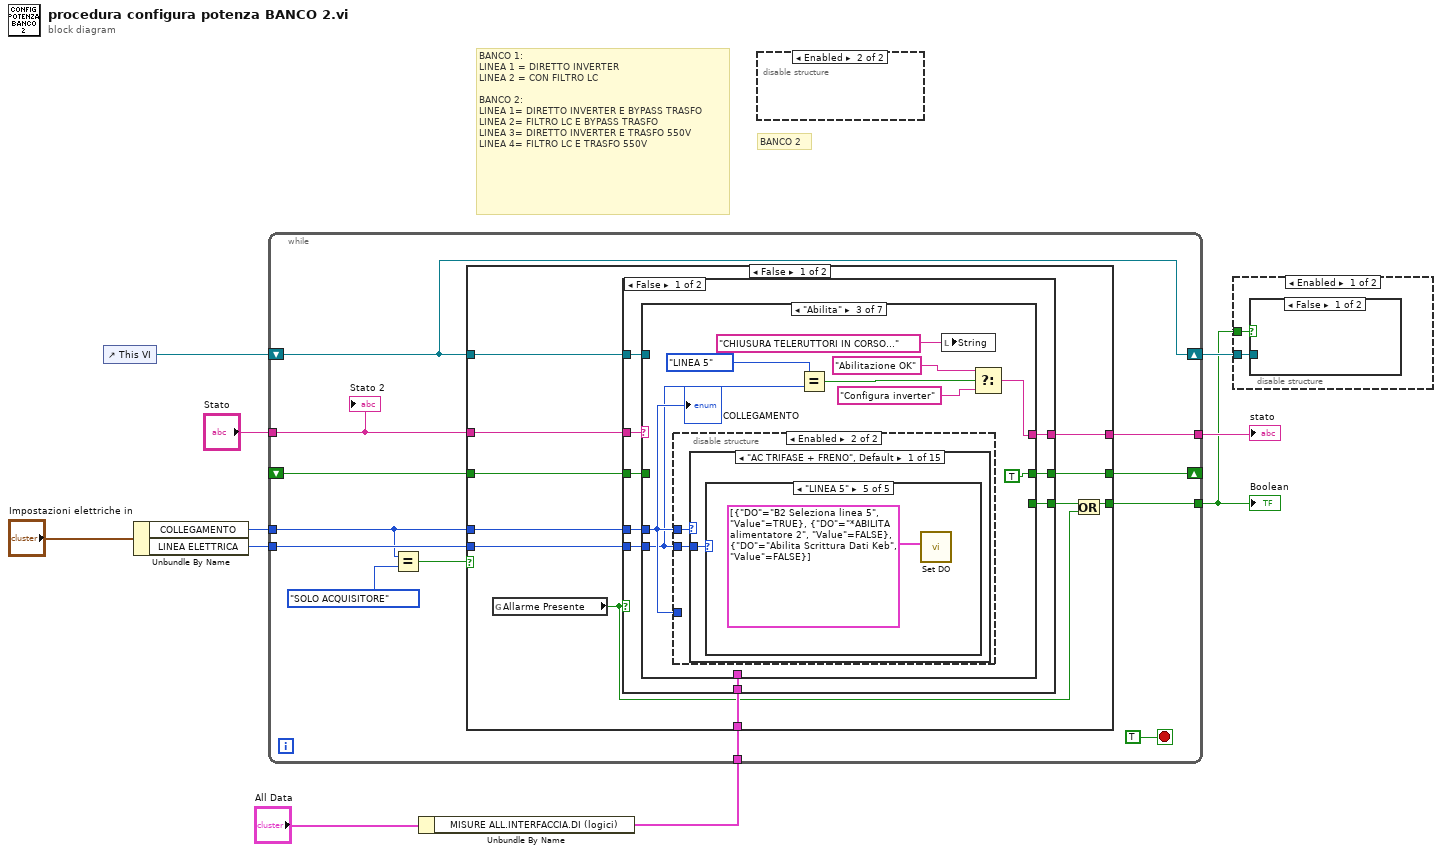
[diagram p0: block diagram]
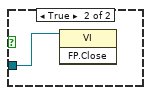
[diagram p2: hidden frame]
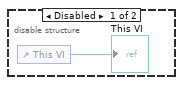
[diagram p4: hidden frame]
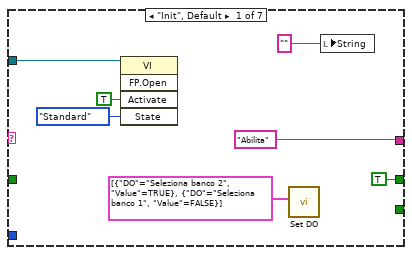
[diagram p5: hidden frame]
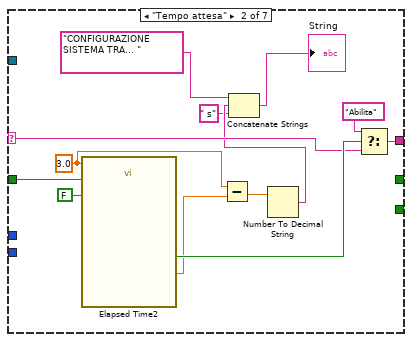
[diagram p6: hidden frame]
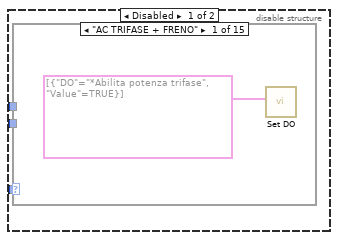
[diagram p7: hidden frame]
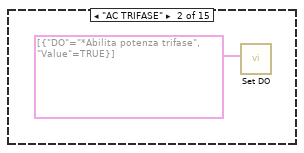
[diagram p8: hidden frame]
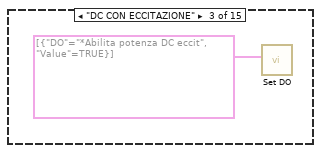
[diagram p9: hidden frame]
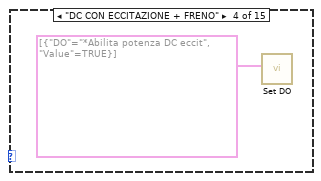
[diagram p10: hidden frame]
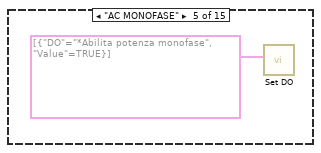
[diagram p11: hidden frame]
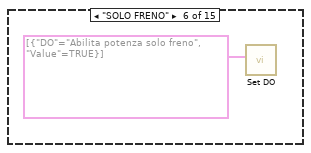
[diagram p12: hidden frame]
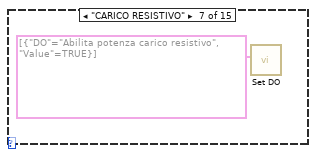
[diagram p13: hidden frame]
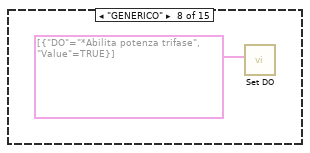
[diagram p14: hidden frame]
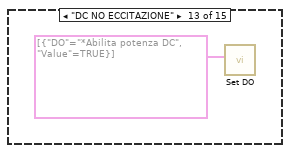
[diagram p19: hidden frame]
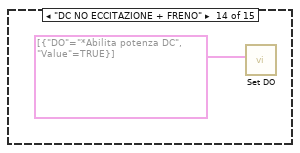
[diagram p20: hidden frame]
diagram:
  # "BANCO 2"
  # "BANCO 1:\nLINEA 1 = DIRETTO INVERTER\nLINEA 2 = CON FILTRO LC\n\nBANCO 2:\nLINEA 1= DIRETTO INVERTER E BYPASS TRASFO\nLINEA 2= FILTRO LC E BYPASS TRASFO\nLINEA 3= DIRETTO INVERTER E TRASFO 550V\nLINEA 4= FILTRO LC E TRASFO 550V"
  n1 = control-ref of="This VI"() -> (w4:refnum<vi>)
  n2 = Unbundle By Name("Impostazioni elettriche in") -> ("COLLEGAMENTO"=w8:T1, "LINEA ELETTRICA"=w3:T30)
  n3 = Unbundle By Name("All Data") -> ("MISURE ALL.INTERFACCIA.DI (logici)"=w9:T31)
  n4 = while {
    shift-right: [w21] -> _
    shift-left: _ -> [w20]
    tunnel: w8 -> [w13]
    tunnel: w9 -> [w19]
    tunnel: [w14] -> w2
    tunnel: "Stato" -> [w18]
    tunnel: [w17] -> w10
    shift-right: [w16] -> w5
    shift-left: w4 -> [w16]
    tunnel: w3 -> [w15]
    stop <- TRUE stop-if-true
    n5 = Equal?(x=w13, y=Collegamenti_elettrici."SOLO ACQUISITORE") -> (x = y?=w11:bool)
    n6 = case shown="False" w11 {
      tunnel: [w33 w237] -> w21
      tunnel: w20 -> [w32 w237]
      tunnel: w19 -> [w31 _]
      tunnel: w18 -> [w29 w235]
      tunnel: [w28 w235] -> w17
      tunnel: w16 -> [w27 _]
      tunnel: w15 -> [w26 _]
      tunnel: [w25 TRUE] -> w14
      tunnel: w13 -> [w23 _]
      frame False {
        n7 = global read "Global allarmi procedure.vi" "Allarme Presente"() -> (w24:bool)
        n8 = case shown="False" w24 {
          tunnel: [w42 _] -> w33
          tunnel: w32 -> [w41 _]
          tunnel: w23 -> [w40 w227]
          tunnel: w31 -> [w39 _]
          tunnel: [w38 TRUE] -> w30
          tunnel: w29 -> [w37 _]
          tunnel: [w36 "Abilitazione KO" ("String")] -> w28
          tunnel: w27 -> [w35 _]
          tunnel: w26 -> [w34 _]
          frame False {
            n9 = case shown="\"Abilita\"" w37 {
              selector: w37 -> [_ w58 _ _ w105 w216 w223]
              tunnel: ["Abilita" ("t") w57 w63 "wait" ("t") w108 w216 w223] -> w36
              tunnel: [TRUE _ TRUE w98 _ _ _] -> w42
              tunnel: w41 -> [_ w62 _ w98 w113 _ _]
              tunnel: w40 -> [_ _ w69 _ w109 _ w220]
              tunnel: w39 -> [_ _ _ _ w110 _ _]
              tunnel: [_ _ _ _ _ TRUE TRUE] -> w38
              tunnel: w35 -> [w48 _ _ _ _ _ _]
              tunnel: w34 -> [_ _ w65 _ w101 _ _]
              frame "Init", Default {
                n10 = invoke class="VI" method="FP.Open"(reference=w48, "Activate"=TRUE ("Activate?"), "State"=T35."Standard") -> ()  [unwired: 2 in, 5 out]
                n11 = call "Set DO.vi"("Cluster SET DO"=T32 [{"DO"=enum."Seleziona banco 2", "Value"=TRUE}, {"DO"=enum."Seleziona banco 1", "Value"=FALSE}]) -> ()  [unwired: 10 in, 1 out]
                n12 = local write "String"("" ("String")) -> ()
              }
              frame "Tempo attesa" {
                w55 = 3.0 ("Time Target (s)")
                n13 = call "Elapsed Time2"("Time Target (s)"=w55, "Reset"=w62, "Auto Reset"=FALSE) -> ("Elapsed Time (s)"=w54:dbl, "Time has Elapsed"=w60:bool)  [unwired: 9 in, 6 out]
                n14 = Subtract(x=w55, y=w54) -> (x-y=w53:dbl)
                n15 = Number To Decimal String(number=w53) -> (decimal integer string=w52:string)  [unwired: 1 in]
                n16 = Concatenate Strings("CONFIGURAZIONE SISTEMA TRA... " ("String"), w52, " s" ("string")) -> (→"String":string)
                n17 = Select(t="Abilita", s=w60, f=w58) -> (s? t:f=w57:string)
              }
              frame "Abilita" {
                n18 = disable-structure shown="Enabled" {
                  disable-tunnel: w69 -> [w72 _]
                  disable-tunnel: w65 -> [_ w85]
                  disable-tunnel: w69 -> [_ w84]
                  frame Disabled {
                    n19 = case shown="\"AC TRIFASE + FRENO\"" w72 {
                      frame "AC TRIFASE + FRENO" {
                        n20 = call "Set DO.vi"("Cluster SET DO"=T32 [{"DO"=enum."*Abilita potenza trifase", "Value"=TRUE}]) -> ()  [unwired: 10 in, 1 out]
                      }
                      frame "AC TRIFASE" {
                        n21 = call "Set DO.vi"("Cluster SET DO"=T32 [{"DO"=enum."*Abilita potenza trifase", "Value"=TRUE}]) -> ()  [unwired: 10 in, 1 out]
                      }
                      frame "DC CON ECCITAZIONE" {
                        n22 = call "Set DO.vi"("Cluster SET DO"=T32 [{"DO"=enum."*Abilita potenza DC eccit", "Value"=TRUE}]) -> ()  [unwired: 10 in, 1 out]
                      }
                      frame "DC CON ECCITAZIONE + FRENO" {
                        n23 = call "Set DO.vi"("Cluster SET DO"=T32 [{"DO"=enum."*Abilita potenza DC eccit", "Value"=TRUE}]) -> ()  [unwired: 10 in, 1 out]
                      }
                      frame "AC MONOFASE" {
                        n24 = call "Set DO.vi"("Cluster SET DO"=T32 [{"DO"=enum."*Abilita potenza monofase", "Value"=TRUE}]) -> ()  [unwired: 10 in, 1 out]
                      }
                      frame "SOLO FRENO" {
                        n25 = call "Set DO.vi"("Cluster SET DO"=T32 [{"DO"=enum."Abilita potenza solo freno", "Value"=TRUE}]) -> ()  [unwired: 10 in, 1 out]
                      }
                      frame "CARICO RESISTIVO" {
                        n26 = call "Set DO.vi"("Cluster SET DO"=T32 [{"DO"=enum."Abilita potenza carico resistivo", "Value"=TRUE}]) -> ()  [unwired: 10 in, 1 out]
                      }
                      frame "GENERICO" {
                        n27 = call "Set DO.vi"("Cluster SET DO"=T32 [{"DO"=enum."*Abilita potenza trifase", "Value"=TRUE}]) -> ()  [unwired: 10 in, 1 out]
                      }
                      frame "SOLO ACQUISITORE" {
                      }
                      frame "SCORTA 4" {
                      }
                      frame "SCORTA 5" {
                      }
                      frame "SCORTA 6" {
                      }
                      frame "DC NO ECCITAZIONE" {
                        n28 = call "Set DO.vi"("Cluster SET DO"=T32 [{"DO"=enum."*Abilita potenza DC", "Value"=TRUE}]) -> ()  [unwired: 10 in, 1 out]
                      }
                      frame "DC NO ECCITAZIONE + FRENO" {
                        n29 = call "Set DO.vi"("Cluster SET DO"=T32 [{"DO"=enum."*Abilita potenza DC", "Value"=TRUE}]) -> ()  [unwired: 10 in, 1 out]
                      }
                      frame "FRENO TRASC + AFE" {
                        n30 = call "Set DO.vi"("Cluster SET DO"=T32 [{"DO"=enum."Abilita AFE + freno trasc", "Value"=TRUE}]) -> ()  [unwired: 10 in, 1 out]
                      }
                    }
                  }
                  frame Enabled {
                    n31 = case shown="\"AC TRIFASE + FRENO\", Default" w84 {
                      tunnel: w85 -> [w86 _ _ _ _ _ _ _ _ _ _ _ _ _ w92]
                      frame "AC TRIFASE + FRENO", Default {
                        n32 = case shown="\"LINEA 5\"" w86 {
                          frame "LINEA 1", Default {
                            n33 = call "Set DO.vi"("Cluster SET DO"=T32 [{"DO"=enum."B2 Seleziona linea 1", "Value"=TRUE}]) -> ()  [unwired: 10 in, 1 out]
                          }
                          frame "LINEA 2" {
                            n34 = call "Set DO.vi"("Cluster SET DO"=T32 [{"DO"=enum."B2 Seleziona linea 2", "Value"=TRUE}]) -> ()  [unwired: 10 in, 1 out]
                          }
                          frame "LINEA 3" {
                            n35 = call "Set DO.vi"("Cluster SET DO"=T32 [{"DO"=enum."B2 Seleziona linea 3", "Value"=TRUE}]) -> ()  [unwired: 10 in, 1 out]
                          }
                          frame "LINEA 4" {
                            n36 = call "Set DO.vi"("Cluster SET DO"=T32 [{"DO"=enum."B2 Seleziona linea 4", "Value"=TRUE}]) -> ()  [unwired: 10 in, 1 out]
                          }
                          frame "LINEA 5" {
                            n37 = call "Set DO.vi"("Cluster SET DO"=T32 [{"DO"=enum."B2 Seleziona linea 5", "Value"=TRUE}, {"DO"=enum."*ABILITA alimentatore 2", "Value"=FALSE}, {"DO"=enum."Abilita Scrittura Dati Keb", "Value"=FALSE}]) -> ()  [unwired: 10 in, 1 out]
                          }
                        }
                      }
                      frame "AC MONOFASE" {
                      }
                      frame "DC CON ECCITAZIONE" {
                      }
                      frame "DC CON ECCITAZIONE + FRENO" {
                      }
                      frame "DC NO ECCITAZIONE" {
                      }
                      frame "DC NO ECCITAZIONE + FRENO" {
                      }
                      frame "FRENO TRASC + AFE" {
                      }
                      frame "SOLO FRENO" {
                      }
                      frame "CARICO RESISTIVO" {
                      }
                      frame "GENERICO" {
                      }
                      frame "SOLO ACQUISITORE" {
                      }
                      frame "SCORTA 4" {
                      }
                      frame "SCORTA 5" {
                      }
                      frame "SCORTA 6" {
                      }
                      frame "AC TRIFASE" {
                        n38 = case shown="\"LINEA 2\"" w92 {
                          frame "LINEA 1", Default {
                            n39 = call "Set DO.vi"("Cluster SET DO"=T32 [{"DO"=enum."B2 Seleziona linea 1", "Value"=TRUE}]) -> ()  [unwired: 10 in, 1 out]
                          }
                          frame "LINEA 2" {
                            n40 = call "Set DO.vi"("Cluster SET DO"=T32 [{"DO"=enum."B2 Seleziona linea 2", "Value"=TRUE}]) -> ()  [unwired: 10 in, 1 out]
                          }
                        }
                      }
                    }
                  }
                }
                n41 = Equal?(x=T30."LINEA 5", y=w65) -> (x = y?=w66:bool)
                n42 = local write "String"("CHIUSURA TELERUTTORI IN CORSO..." ("String")) -> ()
                n43 = Select(t="Abilitazione OK", s=w66, f="Configura inverter") -> (s? t:f=w63:string)
                "COLLEGAMENTO" <- w69
              }
              frame "Configura inverter" {
                n44 = local write "String"("CONFIGURAZIONE INVERTER" ("String")) -> ()
                n45 = call <userlib>:"SMQ_MANAGER.vi"("Function"=enum16{"INITIALIZE", "ENQUEUE", "STOP ALL"}."ENQUEUE", "Queue name"="MAIN_Q", "Enqueue cluster"=T36 {"Array of elements"=[], "Single element"={"String"="CONFIGURA INVERTER", "variant"=variant}, "enque at\nopposite end (F)"=FALSE, "no replications (F)"=FALSE}) -> ()  [unwired: 8 in, 1 out]
              }
              frame "wait" {
                n46 = case shown="\"AC TRIFASE + FRENO\"" w109 {
                  tunnel: [w114 w173 w174 w176 w189 w192 w201 w203 _ _ _ _ w205 w207 w209] -> w102
                  tunnel: w110 -> [w115 w172 w175 w177 w190 w193 w202 w204 _ _ _ _ w206 w208 w210]
                  tunnel: w101 -> [w116 _ _ w178 _ w191 _ _ _ _ _ _ _ _ _]
                  frame "AC TRIFASE + FRENO" {
                    n47 = case shown="\"LINEA 1\", Default" w116 {
                      tunnel: w115 -> [w127 w132 w145 w158 w171]
                      tunnel: [w123 w128 w142 w155 w168] -> w114
                      frame "LINEA 1", Default {
                        n48 = Unbundle By Name(w127) -> ("B2 Scelta linea elettrica 1"=w124:bool, "B2 Scelta linea elettrica 2"=w126:bool, "B2 Scelta linea elettrica 3"=w120:bool, "B2 Scelta linea elettrica 4"=w121:bool, "B2 Scelta linea elettrica 5"=w122:bool)
                        n49 = Not(x=w126) -> (.not. x?=w125:bool)
                        n50 = Not(x=w120) -> (.not. x?=w119:bool)
                        n51 = Not(x=w121) -> (.not. x?=w118:bool)
                        n52 = Not(x=w122) -> (.not. x?=w117:bool)
                        n53 = Compound Arithmetic op=AND(w124, w125, w119, w118, w117) -> (w123:bool)
                      }
                      frame "LINEA 2" {
                        n54 = Unbundle By Name(w132) -> ("B2 Scelta linea elettrica 1"=w131:bool, "B2 Scelta linea elettrica 2"=w129:bool, "B2 Scelta linea elettrica 3"=w136:bool, "B2 Scelta linea elettrica 4"=w137:bool, "B2 Scelta linea elettrica 5"=w138:bool)
                        n55 = Not(x=w136) -> (.not. x?=w135:bool)
                        n56 = Not(x=w137) -> (.not. x?=w134:bool)
                        n57 = Not(x=w138) -> (.not. x?=w133:bool)
                        n58 = Not(x=w131) -> (.not. x?=w130:bool)
                        n59 = Compound Arithmetic op=AND(w130, w129, w135, w134, w133) -> (w128:bool)
                      }
                      frame "LINEA 3" {
                        n60 = Unbundle By Name(w145) -> ("B2 Scelta linea elettrica 1"=w144:bool, "B2 Scelta linea elettrica 2"=w141:bool, "B2 Scelta linea elettrica 3"=w139:bool, "B2 Scelta linea elettrica 4"=w148:bool, "B2 Scelta linea elettrica 5"=w149:bool)
                        n61 = Not(x=w141) -> (.not. x?=w140:bool)
                        n62 = Not(x=w148) -> (.not. x?=w147:bool)
                        n63 = Not(x=w149) -> (.not. x?=w146:bool)
                        n64 = Not(x=w144) -> (.not. x?=w143:bool)
                        n65 = Compound Arithmetic op=AND(w143, w140, w139, w147, w146) -> (w142:bool)
                      }
                      frame "LINEA 4" {
                        n66 = Unbundle By Name(w158) -> ("B2 Scelta linea elettrica 1"=w157:bool, "B2 Scelta linea elettrica 2"=w154:bool, "B2 Scelta linea elettrica 3"=w152:bool, "B2 Scelta linea elettrica 4"=w150:bool, "B2 Scelta linea elettrica 5"=w160:bool)
                        n67 = Not(x=w154) -> (.not. x?=w153:bool)
                        n68 = Not(x=w160) -> (.not. x?=w159:bool)
                        n69 = Not(x=w157) -> (.not. x?=w156:bool)
                        n70 = Not(x=w152) -> (.not. x?=w151:bool)
                        n71 = Compound Arithmetic op=AND(w156, w153, w151, w150, w159) -> (w155:bool)
                      }
                      frame "LINEA 5" {
                        n72 = Unbundle By Name(w171) -> ("B2 Scelta linea elettrica 1"=w170:bool, "B2 Scelta linea elettrica 2"=w167:bool, "B2 Scelta linea elettrica 3"=w165:bool, "B2 Scelta linea elettrica 4"=w163:bool, "B2 Scelta linea elettrica 5"=w161:bool)
                        n73 = Not(x=w167) -> (.not. x?=w166:bool)
                        n74 = Not(x=w170) -> (.not. x?=w169:bool)
                        n75 = Not(x=w165) -> (.not. x?=w164:bool)
                        n76 = Not(x=w163) -> (.not. x?=w162:bool)
                        n77 = Compound Arithmetic op=AND(w169, w166, w164, w162, w161) -> (w168:bool)
                      }
                    }
                  }
                  frame "DC CON ECCITAZIONE" {
                    n78 = Unbundle By Name(w172) -> ("Potenza DC ECC abilitata"=w173:bool)
                  }
                  frame "DC CON ECCITAZIONE + FRENO" {
                    n79 = Unbundle By Name(w175) -> ("Potenza DC ECC abilitata"=w174:bool)
                  }
                  frame "AC TRIFASE" {
                    n80 = case shown="\"LINEA 2\"" w178 {
                      tunnel: w177 -> [w183 w185]
                      tunnel: [w179 w184] -> w176
                      frame "LINEA 1", Default {
                        n81 = Unbundle By Name(w183) -> ("B2 Scelta linea elettrica 1"=w180:bool, "B2 Scelta linea elettrica 2"=w182:bool)
                        n82 = Not(x=w182) -> (.not. x?=w181:bool)
                        n83 = And(x=w180, y=w181) -> (x .and. y?=w179:bool)
                      }
                      frame "LINEA 2" {
                        n84 = Unbundle By Name(w185) -> ("B2 Scelta linea elettrica 2"=w186:bool, "B2 Scelta linea elettrica 1"=w188:bool)
                        n85 = Not(x=w188) -> (.not. x?=w187:bool)
                        n86 = And(x=w186, y=w187) -> (x .and. y?=w184:bool)
                      }
                    }
                  }
                  frame "AC MONOFASE" {
                    n87 = Unbundle By Name(w190) -> ("Potenza monofase abilitata"=w189:bool)
                  }
                  frame "SOLO FRENO" {
                    n88 = disable-structure shown="Enabled" {
                      disable-tunnel: w193 -> [w196 _]
                      disable-tunnel: [w194 TRUE] -> w192
                      disable-tunnel: w191 -> [_ _]
                      frame Disabled {
                        n89 = Unbundle By Name(w196) -> ("B2 Scelta linea elettrica 2"=w197:bool, "B2 Scelta linea elettrica 1"=w199:bool)
                        n90 = Not(x=w197) -> (.not. x?=w195:bool)
                        n91 = Not(x=w199) -> (.not. x?=w198:bool)
                        n92 = And(x=w195, y=w198) -> (x .and. y?=w194:bool)
                      }
                      frame Enabled {
                      }
                    }
                  }
                  frame "CARICO RESISTIVO" {
                    n93 = Unbundle By Name(w202) -> ("DI (logici) aggiuntivi impianto.Carico resistivo abilitato"=w201:bool)
                  }
                  frame "GENERICO" {
                    n94 = Unbundle By Name(w204) -> ("Potenza trifase abilitata"=w203:bool)
                  }
                  frame "SOLO ACQUISITORE" {
                  }
                  frame "SCORTA 4" {
                  }
                  frame "SCORTA 5" {
                  }
                  frame "SCORTA 6" {
                  }
                  frame "DC NO ECCITAZIONE" {
                    n95 = Unbundle By Name(w206) -> ("Potenza DC abilitata"=w205:bool)
                  }
                  frame "DC NO ECCITAZIONE + FRENO" {
                    n96 = Unbundle By Name(w208) -> ("Potenza DC abilitata"=w207:bool)
                  }
                  frame "FRENO TRASC + AFE" {
                    n97 = Unbundle By Name(w210) -> ("DI (logici) aggiuntivi impianto.AFE+freno abilitato"=w209:bool)
                  }
                }
                n98 = call "Elapsed Time"("Time Target (s)"=5.0, "Reset"=w113, "Auto Reset"=FALSE) -> ("Time has Elapsed"=w106:bool)  [unwired: 9 in, 7 out]
                n99 = Select(t="Abilitazione KO", s=w106, f=w105) -> (s? t:f=w104:string)
                n100 = Select(t="Abilitazione OK", s=w102, f=w104) -> (s? t:f=w108:string)
              }
              frame "Abilitazione OK" {
                n101 = Wait (ms)(milliseconds to wait=u32 1000) -> ()  [unwired: 1 out]
                n102 = call <userlib>:"SMQ_MANAGER.vi"("Function"=enum16{"INITIALIZE", "ENQUEUE", "STOP ALL"}."ENQUEUE", "Queue name"="MAIN_Q", "Enqueue cluster"=T36 {"Array of elements"=[], "Single element"={"String"="POTENZA ABILITATA", "variant"=variant}, "enque at\nopposite end (F)"=FALSE, "no replications (F)"=FALSE}) -> ()  [unwired: 8 in, 1 out]
                n103 = local write "String"("ABILITAZIONE OK. FINE" ("String")) -> ()
              }
              frame "Abilitazione KO" {
                n104 = Wait (ms)(milliseconds to wait=u32 1000) -> ()  [unwired: 1 out]
                n105 = case shown="\"AC TRIFASE\", Default" w220 {
                  frame "AC TRIFASE", Default {
                    n106 = global write "Global allarmi procedure.vi" "Allarme Abilita potenza"(TRUE ("Allarme Abilita potenza")) -> ()
                  }
                  frame "CARICO RESISTIVO" {
                    n107 = global write "Global allarmi procedure.vi" "carico resistivo non trovato"(TRUE ("Allarme Abilita potenza")) -> ()
                  }
                }
                n108 = local write "String"("ABILITAZIONE KO. FINE" ("String")) -> ()
                n109 = call "Set DO.vi"("Cluster SET DO"=T32 [{"DO"=enum."*Disabilita teleruttori potenza", "Value"=TRUE}]) -> ()  [unwired: 10 in, 1 out]
              }
            }
          }
          frame True {
            n110 = case shown="\"CARICO RESISTIVO\"" w227 {
              frame "AC TRIFASE", Default {
                n111 = global write "Global allarmi procedure.vi" "Allarme Abilita potenza"(TRUE ("Allarme Abilita potenza")) -> ()
              }
              frame "CARICO RESISTIVO" {
                n112 = global write "Global allarmi procedure.vi" "carico resistivo non trovato"(TRUE ("Allarme Abilita potenza")) -> ()
              }
            }
            n113 = Wait (ms)(milliseconds to wait=u32 1000) -> ()  [unwired: 1 out]
            n114 = local write "String"("ABILITAZIONE KO. FINE" ("String")) -> ()
            n115 = call "Set DO.vi"("Cluster SET DO"=T32 [{"DO"=enum."*Disabilita teleruttori potenza", "Value"=TRUE}]) -> ()  [unwired: 10 in, 1 out]
          }
        }
        n116 = Or(x=w30, y=w24) -> (x .or. y?=w25:bool)
      }
      frame True {
        # "MODALITà SOLO ACQUISITORE SCEGLI SOLO IL BANCO\nPER LA LETTURA DEL TORSIOMETRO CORRETTO E \nNON FARE ALTRO (ANCHE IN CASO DI ALLARME PRESENTE\nO QUADRI DI POTENZA SPENTI)"
        n117 = flat-sequence {
          frame #0 {
            n118 = call "Set DO.vi"("Cluster SET DO"=T32 [{"DO"=enum."Seleziona banco 2", "Value"=TRUE}, {"DO"=enum."Seleziona banco 1", "Value"=FALSE}]) -> ()  [unwired: 10 in, 1 out]
          }
          frame #1 {
            n119 = Wait (ms)(milliseconds to wait=u32 1500) -> ()  [unwired: 1 out]
          }
        }
        n120 = local write "String"("SCELTA BANCO 2 (KEB).. OK" ("String")) -> ()
      }
    }
    "Stato 2" <- w18
  }
  "stato" <- w10
  "Boolean" <- w2
  n121 = disable-structure shown="Enabled" {
    frame Disabled {
      n122 = control-ref of="This VI"() -> (→"This VI":refnum<vi>)
    }
    frame Enabled {
    }
  }
  n123 = disable-structure shown="Enabled" {
    disable-tunnel: w2 -> [w242 _]
    disable-tunnel: w5 -> [w241 _]
    frame Enabled {
      n124 = case shown="False" w242 {
        tunnel: w241 -> [_ w243]
        frame False {
        }
        frame True {
          n125 = invoke class="VI" method="FP.Close"(reference=w243) -> ()  [unwired: 2 in, 3 out]
        }
      }
    }
    frame Disabled {
    }
  }
